vi "Shore Remote.vi"() -> ()   [LabVIEW 2015, in "Shore Library.lvlib"]
uses:
  Shore Library.lvlib
  Libraries/RDS Instruments/Battery/Battery Data.ctl
  Libraries/RDS Child Messages/Battery Data/Battery Status.ctl
  Libraries/RDS Instruments/AIP/AIP Status.ctl
  Libraries/RDS Instruments/AIP/AIP States.ctl
  Libraries/RDS Child Messages/Depth Data Message/Depth Data.ctl
  Libraries/RDS Child Messages/Helm/Helm Status Message/Helm Status Control.ctl
  Actors/RDS Helm Actor/RDS Helm Actor/Helm State.ctl
  Libraries/RDS Child Messages/Helm/Heading Command/Heading Command Cntrl.ctl
  Libraries/RDS Child Messages/Helm/Steering Command/Steering Command Cntrl.ctl
  Libraries/RDS Child Messages/PID Gains/PID Gains Control.ctl
  Libraries/RDS Child Messages/Mission Messages/Mission Controller State Control.ctl
  RDS Mission Controller Actor/Mission Controller Navigation State.ctl
  RDS Mission Controller Actor/MissionOp.ctl
  Libraries/RDS Child Messages/MCB/MCB Motor Status.ctl
  Libraries/RDS Instruments/Compass/Compass Data.ctl
  Libraries/3rd Party/NMEA_GPS/NMEA_GPRMC-data.ctl
  Libraries/3rd Party/NMEA_GPS/NMEA_LatitudeDirection.ctl
  Libraries/3rd Party/NMEA_GPS/NMEA_LongitudeDirection.ctl
  Libraries/RDS Serial Handler/RDS Serial Instrument.lvclass
  RDS State Tracker/RDS State/RDS State.lvclass
  Libraries/RDS Serial Handler/RDS Serial Frame.lvclass/RDS Serial Frame.ctl
  Libraries/RDS Serial Handler/RDS Serial Frame.lvclass
  Libraries/RDS Serial Handler/RDS Serial Instrument.lvclass/RDS Serial Instrument.ctl
  RDS State Tracker/RDS State/RDS State.lvclass/RDS State.ctl
  <vilib>/Utility/inputDevices.llb/joystickAcquire.vi
  <vilib>/Utility/inputDevices.llb/closeJoystick.vi
  Libraries/RDS Child Messages/RDS Child Messages.lvlib
  Libraries/Geo/RDS Libraries.lvlib
  LSR Instrument Actor/LSR Instrument/LSR Instrument.lvlib
  Libraries/RDS Instruments/RDS Instrument Library.lvlib
  Actors/RDS Helm Actor/RDS Helm Actor.lvlib
  RDS Mission Controller Actor/RDS Mission Controller Actor.lvlib
  Libraries/RDS Child Messages/Mission Messages/Mission Controller State Message.lvclass
  Libraries/3rd Party/NMEA_GPS/NMEA.lvlib
panel:
  out "length":i32
  out "length 2":i32
  out "Time Stamp":timestamp
  in  "Boolean":bool=TRUE
  in  "Tab Control":T1(tab)
  out "LSR Connected":bool
  out "output cluster":T2
  in  "Joystick!":bool
  in  "Rudder":i8
  in  "Throttle":i16
  out "Battery Pack Info":T3
  out "AIP Status":T5
  out "Depth Data":T7
  out "Compass Data":T8
  out "GPRMC-data":T9={"TimeStamp"=timestamp(0 s since 1904-01-01), "Validity"=FALSE, "Latitude"=0.0, "Latitude-Direction"=enum."North", "Longitude"=0.0, "Longitude-Direction"=enum."East", "Speed in knots"=0.0, "True course"=0.0, "Date Stamp"=timestamp(0 s since 1904-01-01), "Magnetic Variation (East/West)"=0.0, "GPS Latitude"=0.0, "GPS Longitude"=0.0} {"GPS Longitude" format="%.6f"; "GPS Latitude" format="%.6f"; "Magnetic Variation (East/West)" format="%.02f [deg]"; "Date Stamp" format="%<%x>T"; "True course" format="%.02f [deg]"; "Speed in knots" format="%.02f [kts]"; "Longitude" format="%0.4f [long]"; "Latitude" format="%.04f [lat]"; "TimeStamp" format="%<%.2X>T"}
  out "Helm Status":T12 {"Gains"."D (Td)" format="%#_9f"; "Gains"."I (Ti)" format="%#_9f"; "Gains"."P (Kc)" format="%#.9f"}
  out "Mission Controller State":T16 {"Mission"."GPS Longitude" format="%.6g"; "Mission"."GPS Latitude" format="%.6g"}
  out "Port Motor Data":T19
  out "STBD Motor":T19
  in  "stop":bool
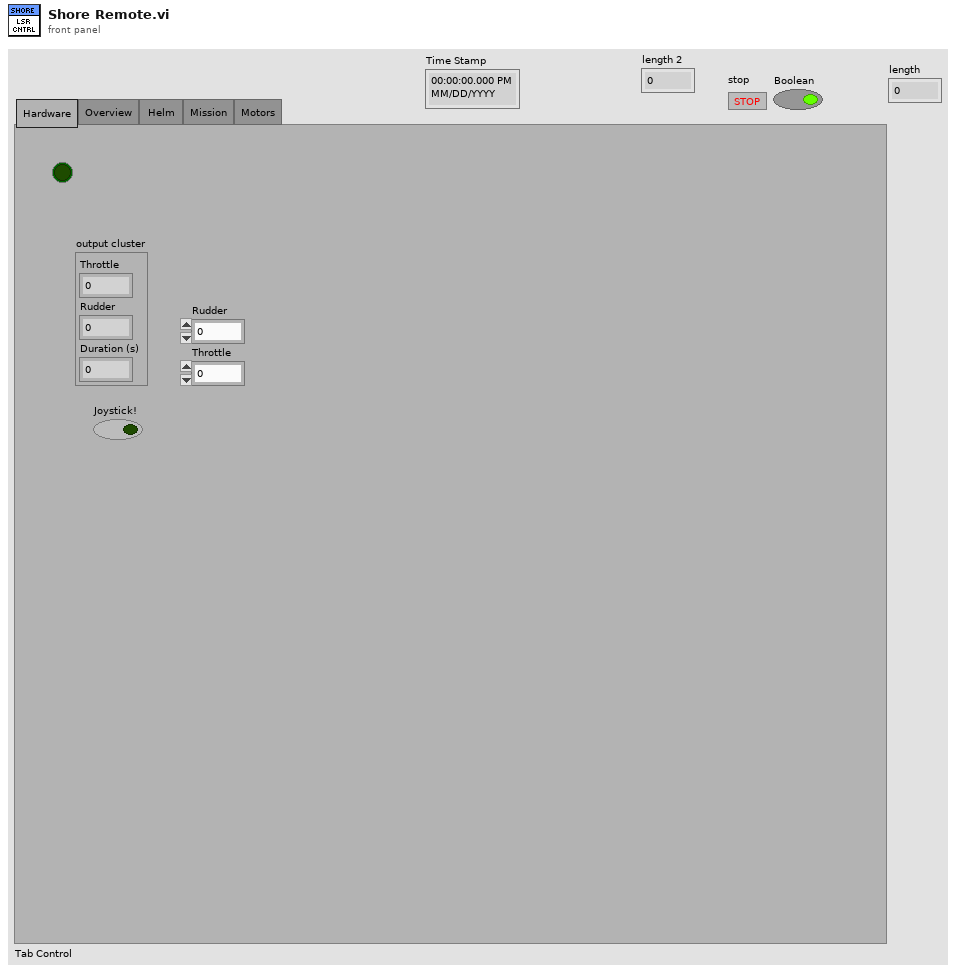
[diagram p1: front panel]
types:
  T1 = enum32{"Hardware", "Overview", "Helm ", "Mission", "Motors"}
  T2 = typedef "RDS Child Messages.lvlib/Steering Command Cntrl.ctl" = cluster{"Throttle":i16, "Rudder":i8, "Duration (s)":u16}
  T3 = typedef "RDS Instrument Library.lvlib/Battery Data.ctl" = cluster{"Battery Status":T4, "Pack Voltage":sgl, "Pack Current":sgl, "Pack Capacity":sgl, "Max Cell Temp":sgl, "Min Cell Temp":sgl, "Max Cell Voltage":sgl, "Min Cell Voltage":sgl}
  T4 = typedef "RDS Instrument Library.lvlib/Battery Status.ctl" = enum16{"Pack Normal", "Alarm: Cell temp too high", "Alarm: Pack voltage too high", "Warn: Pack voltage too high ", "Alarm: Pack voltage too low", "Warn: Pack voltage low", "Alarm Pack current too high", "Warn: Pack current too high ", "Fault: Pack to chassis connection detected", "Fault: Pack to cell connection error", "Fautl: System error"}
  T5 = typedef "RDS Instrument Library.lvlib/AIP Status.ctl" = cluster{"FWD Port":T6, "FWD Stbd":T6, "AFT Port":T6, "AFT Stbd":T6}
  T6 = typedef "RDS Instrument Library.lvlib/AIP States.ctl" = enum16{"Deploy", "Deploying", "Deployed", "Stow", "Stowing", "Stowed", "Fault", "brakeOnStow", "breakOnDeploy", "Stopped", "Stopping"}
  T7 = typedef "RDS Child Messages.lvlib/Depth Data.ctl" = cluster{"Depth":sgl, "Water Temp":i8}
  T8 = typedef "RDS Instrument Library.lvlib/Compass Data.ctl" = cluster{"Compass Heading":sgl, "pitch Angle":sgl, "roll Angle":sgl, "Temperature":sgl, "Depth":sgl, "Magnetic Field":sgl, "Magnetic Field X":sgl, "Magnetic Field Y":sgl, "Magnetic Field Z":sgl, "Acceleration":sgl, "Acceleration X":sgl, "Acceleration Y":sgl, "Gyro":sgl, "Gyro X":sgl, "Acceleration Z":sgl, "Gyro Y":sgl, "Raw Heading":sgl}
  T9 = typedef "RDS Libraries.lvlib/NMEA.lvlib/NMEA_GPRMC-data.ctl" = cluster{"TimeStamp":timestamp, "Validity":bool, "Latitude":dbl, "Latitude-Direction":T10, "Longitude":dbl, "Longitude-Direction":T11, "Speed in knots":sgl, "True course":sgl, "Date Stamp":timestamp, "Magnetic Variation (East/West)":sgl, "GPS Latitude":dbl, "GPS Longitude":dbl}
  T10 = typedef "RDS Libraries.lvlib/NMEA.lvlib/NMEA_LatitudeDirection.ctl" = enum16{"", "North", "South"}
  T11 = typedef "RDS Libraries.lvlib/NMEA.lvlib/NMEA_LongitudeDirection.ctl" = enum16{"", "East", "West"}
  T12 = typedef "RDS Child Messages.lvlib/Helm Status Control.ctl" = cluster{"Helm State":T13, "Heading Command Control":T14, "Steering Command Control":T2, "Last Command Time":timestamp, "Gains":T15, "Current Heading":dbl, "Port Throttle":i16, "STBD Throttle":i16, "Limiter":dbl}
  T13 = typedef "RDS Helm Actor.lvlib/Helm State.ctl" = enum16{"Idle", "Executing Heading Command", "Executing Steering Command"}
  T14 = typedef "RDS Child Messages.lvlib/Heading Command Cntrl.ctl" = cluster{"Throttle":i16, "Heading":sgl, "Duration (s)":i16}
  T15 = typedef "RDS Child Messages.lvlib/PID Gains Control.ctl" = cluster{"P (Kc)":sgl, "I (Ti)":sgl, "D (Td)":sgl}
  T16 = typedef "RDS Child Messages.lvlib/Mission Controller State Message.lvclass/Mission Controller State Control.ctl" = cluster{"iHasControl":bool, "controlTimer":timestamp, "Nav State":T17, "Current MissionOp Index":i32, "Mission":T18[], "Distance to Target":dbl, "Seconds to Timeout":dbl}
  T17 = typedef "RDS Mission Controller Actor.lvlib/Mission Controller Navigation State.ctl" = cluster{"GPS Latitude":ext, "GPS Longitude":ext, "Compass Heading":dbl, "Speed":dbl}
  T18 = typedef "RDS Mission Controller Actor.lvlib/MissionOp.ctl" = cluster{"MissionOp Type":enum16{"Waypoint", "Loiter", "Wait", "Deploy AIP", "Stow AIP"}, "Duration (s)":u16, "Throttle":i16, "GPS Latitude":dbl, "GPS Longitude":dbl, "Loiter Range (m)":u16}
  T19 = typedef "RDS Child Messages.lvlib/MCB Motor Status.ctl" = cluster{"Motor Power":i16, "Motor Command":i16, "Battery Volts":sgl, "Battery Amps":sgl, "Motor Amps":sgl, "MCU Temp":i16, "Heatsink Temp":i16, "Fault Flags":u16, "StatusFlags":u16}
  T20 = cluster{"X axis":i32, "Y axis":i32, "Z axis":i32, "X axis rotation":i32, "Y axis rotation":i32, "Z axis rotation":i32, "U axis":i32, "V axis":i32}
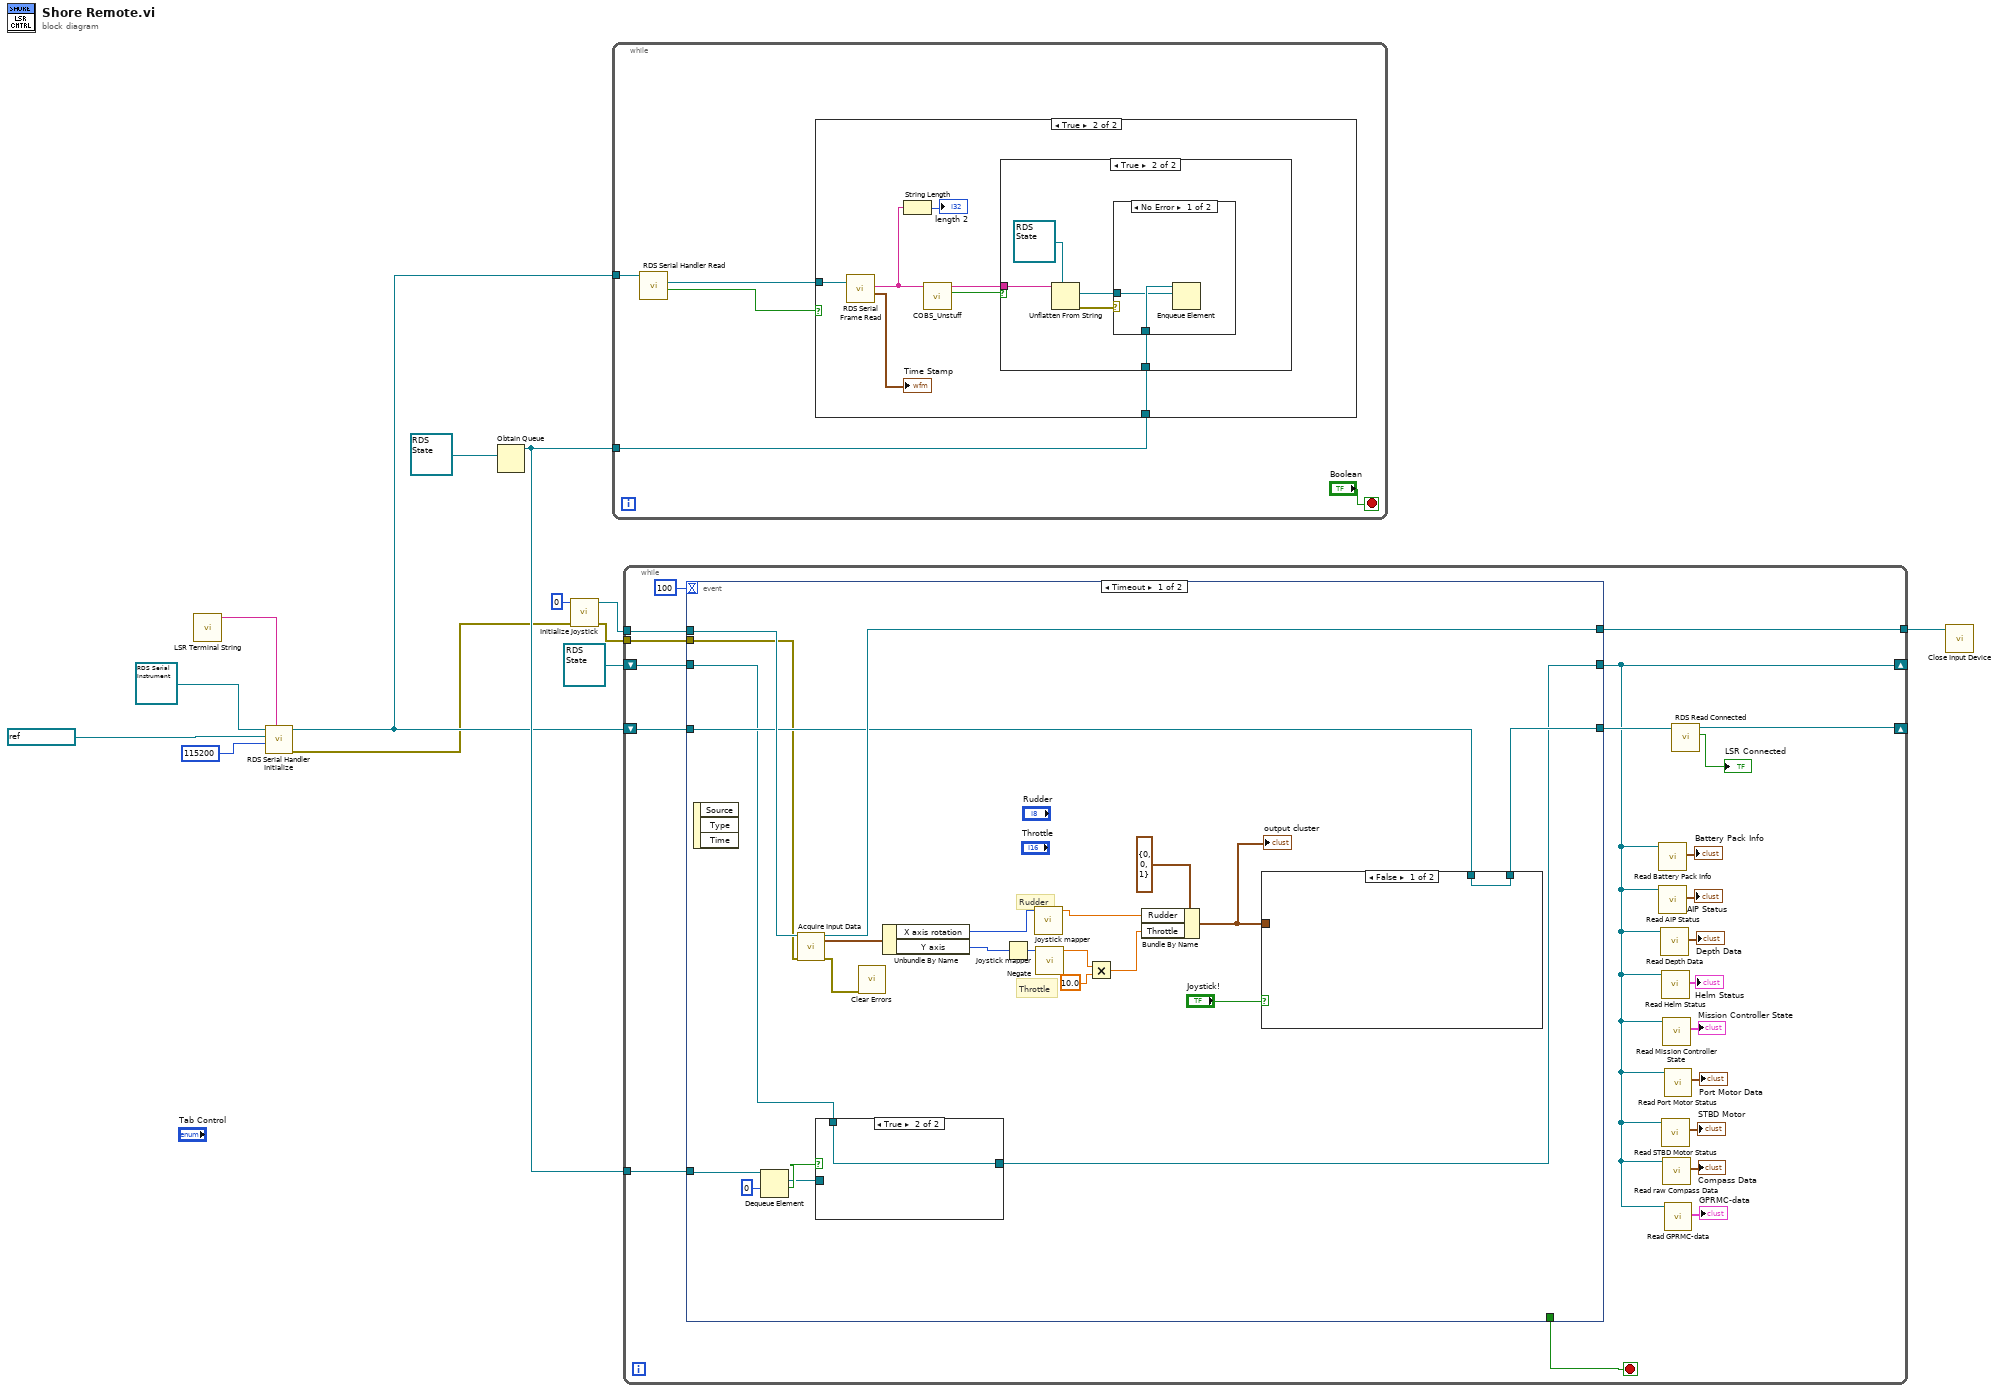
[diagram p0: block diagram]
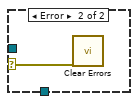
[diagram p4: hidden frame]
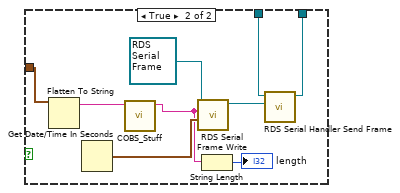
[diagram p5: hidden frame]
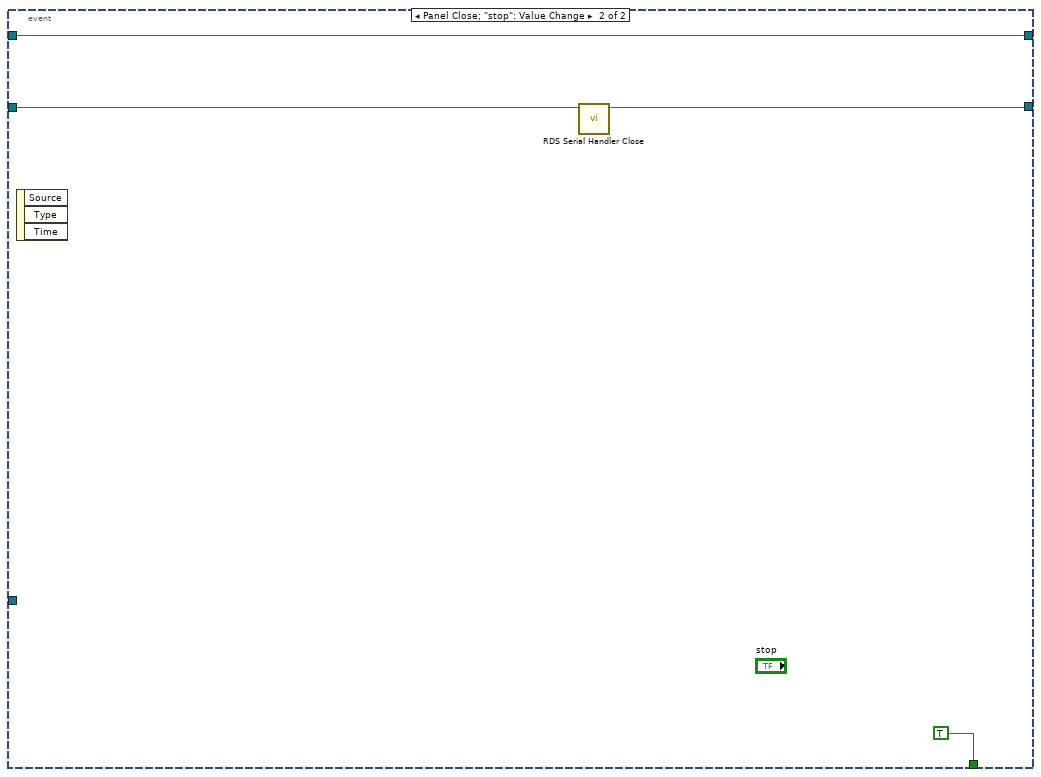
[diagram p7: hidden frame]
diagram:
  n1 = call "LSR Terminal String.vi"() -> ("LSR Term"=w10:string)  [unwired: 11 in]
  n2 = call "RDS Serial Handler Initialize.vi"("Termination Char(s)"=w10, "baud rate (9600)"=u32 115200, "VISA resource name"=refnum<visa-resource-name> "COM11", "RDS Serial Instrument in"=refnum<class "RDS Serial Instrument.lvclass"> refnum ("RDS Serial Handler.lvlib:RDS Serial Instrument.lvclass")) -> ("error out"=w1:errorcluster, "RDS Serial Instrument out"=w5:refnum<class "RDS Serial Instrument.lvclass">)  [unwired: 6 in]
  n3 = Obtain Queue(element data type=refnum<class "RDS State.lvclass"> refnum ("RDS Child Messages.lvlib:RDS State.lvclass")) -> (queue out=w11:refnum<queue>)  [unwired: 4 in, 2 out]
  n4 = call <vilib>:"Initialize Joystick.vi"("error in (no error)"=w1, "device index"=0) -> ("error out"=w2:errorcluster, "device ID"=w7:refnum<k1>)  [unwired: 8 in]
  n5 = while {
    tunnel: w11 -> [w14]
    tunnel: w5 -> [w15]
    stop <- "Boolean" stop-if-true
    n6 = call "RDS Serial Handler Read.vi"("RDS Serial Instrument in"=w15) -> ("Data Valid?"=w16:bool, "RDS Serial Frame out"=w17:refnum<class "RDS Serial Frame.lvclass">)  [unwired: 7 in, 2 out]
    n7 = case shown="True" w16 {
      tunnel: w17 -> [_ w25]
      tunnel: w14 -> [_ w22]
      frame False {
      }
      frame True {
        n8 = call "RDS Serial Frame Read.vi"("RDS Serial Frame in"=w25) -> ("Time Stamp"=→"Time Stamp":timestamp, "Serial String"=w21:string)  [unwired: 7 in, 2 out]
        n9 = String Length(string=w21) -> (length=→"length 2":i32)
        n10 = call "COBS_Unstuff.vi"("Suffed data"=w21) -> ("Valid?"=w19:bool, "Unstuffed String"=w20:string)  [unwired: 8 in, 1 out]
        n11 = case shown="True" w19 {
          tunnel: w22 -> [_ w27]
          tunnel: w20 -> [_ w26]
          frame False {
          }
          frame True {
            n12 = Unflatten From String(type=refnum<class "RDS State.lvclass"> refnum ("RDS Child Messages.lvlib:RDS State.lvclass"), binary string=w26) -> (value=w30:refnum<class "RDS State.lvclass">, error out=w29:errorcluster)  [unwired: 3 in, 1 out]
            n13 = case shown="No Error" w29 {
              selector: w29 -> [_ w33]
              tunnel: w30 -> [w31 _]
              tunnel: w27 -> [w32 _]
              frame No Error {
                n14 = Enqueue Element(queue=w32, element=w31) -> ()  [unwired: 2 in, 3 out]
              }
              frame Error {
                n15 = call <vilib>:"Clear Errors.vi"("error in (no error)"=w33) -> ()  [unwired: 5 in, 2 out]
              }
            }
          }
        }
      }
    }
  }
  n16 = while {
    shift-right: [w51] -> _
    shift-left: w5 -> [w53]
    shift-right: [w47] -> _
    shift-left: refnum<class "RDS State.lvclass"> refnum ("RDS Child Messages.lvlib:RDS State.lvclass") -> [w48]
    tunnel: w11 -> [w37]
    tunnel: w7 -> [w36]
    tunnel: [w35] -> w6
    tunnel: w2 -> [w34]
    stop <- w54 stop-if-true
    n17 = event shown="[0] Timeout" {
      selector: _ -> [_ _]
      dyn-events: _ -> [_ _]
      timeout: 100 -> [_ _]
      tunnel: [_ TRUE] -> w54
      tunnel: [w66 w91] -> w52
      tunnel: w53 -> [w67 w92]
      tunnel: w48 -> [w62 w90]
      tunnel: [w61 w90] -> w47
      tunnel: w37 -> [w65 _]
      tunnel: w36 -> [w70 _]
      tunnel: [w69 _] -> w35
      tunnel: w34 -> [w58 _]
      event Timeout {
        # "Throttle"
        # "Rudder"
        n18 = event-data() -> ()  [unwired: 1 in, 3 out]
        n19 = Dequeue Element(queue=w65, timeout in ms (-1)=0) -> (element=w60:refnum<class "RDS State.lvclass">, timed out?=w63:bool)  [unwired: 1 in, 2 out]
        n20 = call-poly <vilib>:"Acquire Input Data.vi"("device ID"=w70, "error in (no error)"=w58) -> ("device ID"=w69:refnum<k1>, "axis info"=w71:T20, "error out"=w57:errorcluster)  [unwired: 15 out]
        n21 = case shown="True" w63 {
          tunnel: [w88 w89] -> w61
          tunnel: w62 -> [_ w89]
          tunnel: w60 -> [w88 _]
          frame False {
          }
          frame True {
          }
        }
        n22 = call <vilib>:"Clear Errors.vi"("error in (no error)"=w57) -> ()  [unwired: 5 in, 2 out]
        n23 = Unbundle By Name(w71) -> ("X axis rotation"=w75:i32, "Y axis"=w76:i32)
        n24 = Negate(x=w76) -> (-x=w72:i32)
        n25 = call "Joystick mapper.vi"("Input"=w75) -> ("Output"=w56:dbl)  [unwired: 10 in]
        n26 = call "Joystick mapper.vi"("Input"=w72) -> ("Output"=w74:dbl)  [unwired: 10 in]
        n27 = Multiply(x=w74, y=10.0) -> (x*y=w55:dbl)
        n28 = Bundle By Name(cluster=T2 {"Throttle"=0, "Rudder"=0, "Duration (s)"=1} ("Steering Command Control"), "Rudder"=w56, "Throttle"=w55) -> (w68:T2)
        "output cluster" <- w68
        n29 = case shown="False" "Joystick!" {
          tunnel: w68 -> [_ w85]
          tunnel: w67 -> [w78 w84]
          tunnel: [w78 w83] -> w66
          frame False {
          }
          frame True {
            n30 = Flatten To String(anything=w85) -> (data string=w80:string)  [unwired: 3 in, 2 out]
            n31 = Get Date/Time In Seconds() -> (seconds since 1Jan1904=w81:timestamp)
            n32 = call "COBS_Stuff.vi"("Raw data"=w80) -> ("Stuffed Data"=w79:string)  [unwired: 9 in, 1 out]
            n33 = call "RDS Serial Frame Write.vi"("Time Stamp"=w81, "Serial String"=w79, "RDS Serial Frame in"=refnum<class "RDS Serial Frame.lvclass"> refnum) -> ("RDS Serial Frame out"=w87:refnum<class "RDS Serial Frame.lvclass">)  [unwired: 7 in, 1 out]
            n34 = String Length(string=w79) -> (length=→"length":i32)
            n35 = call "RDS Serial Handler Send Frame.vi"("Serial Frame"=w87, "RDS Serial Instrument in"=w84) -> ("RDS Serial Instrument out"=w83:refnum<class "RDS Serial Instrument.lvclass">)  [unwired: 8 in, 1 out]
          }
        }
      }
      event Panel Close; "stop": Value Change {
        n36 = event-data() -> ()  [unwired: 1 in, 3 out]
        n37 = call "RDS Serial Handler Close.vi"("RDS Serial Instrument in"=w92) -> ("RDS Serial Instrument out"=w91:refnum<class "RDS Serial Instrument.lvclass">)  [unwired: 9 in, 1 out]
      }
    }
    n38 = call "Read Battery Pack Info.vi"("RDS State in"=w47) -> ("Battery Pack Info"=→"Battery Pack Info":T3)  [unwired: 8 in, 2 out]
    n39 = call "Read AIP Status.vi"("RDS State in"=w47) -> ("AIP Status"=→"AIP Status":T5)  [unwired: 8 in, 2 out]
    n40 = call "Read Depth Data.vi"("RDS State in"=w47) -> ("Depth Data"=→"Depth Data":T7)  [unwired: 8 in, 2 out]
    n41 = call "Read Helm Status.vi"("RDS State in"=w47) -> ("Helm Status"=→"Helm Status":T12)  [unwired: 8 in, 2 out]
    n42 = call "Read STBD Motor Status.vi"("RDS State in"=w47) -> ("STBD Motor"=→"STBD Motor":T19)  [unwired: 8 in, 2 out]
    n43 = call "Read Mission Controller State.vi"("RDS State in"=w47) -> ("Mission Controller State"=→"Mission Controller State":T16)  [unwired: 8 in, 2 out]
    n44 = call "Read raw Compass Data.vi"("RDS State in"=w47) -> ("Compass Data"=→"Compass Data":T8)  [unwired: 8 in, 2 out]
    n45 = call "Read Port Motor Status.vi"("RDS State in"=w47) -> ("Port Motor Data"=→"Port Motor Data":T19)  [unwired: 8 in, 2 out]
    n46 = call "Read GPRMC-data.vi"("RDS State in"=w47) -> ("GPRMC-data"=→"GPRMC-data":T9)  [unwired: 8 in, 2 out]
    n47 = call "RDS Read Connected.vi"("RDS Serial Instrument in"=w52) -> ("Connected"=→"LSR Connected":bool, "RDS Serial Instrument out"=w51:refnum<class "RDS Serial Instrument.lvclass">)  [unwired: 8 in, 1 out]
  }
  n48 = call-poly <vilib>:"Close Input Device.vi"("device ID"=w6) -> ()  [unwired: 9 in, 1 out]
